vi "MakeArray.vi"(6 "Hviletid(s)":dbl, 9 "Amplitude(kPA)":dbl, 10 "Frekvens(kHz)":dbl, 11 "Temperatur(Celsius)":dbl) -> (3 "Array":dbl[](array[numeric]))   [LabVIEW 2015]
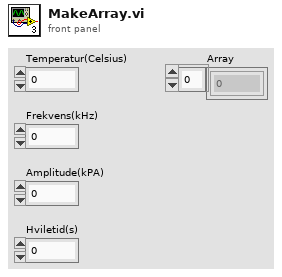
[diagram p1: front panel]
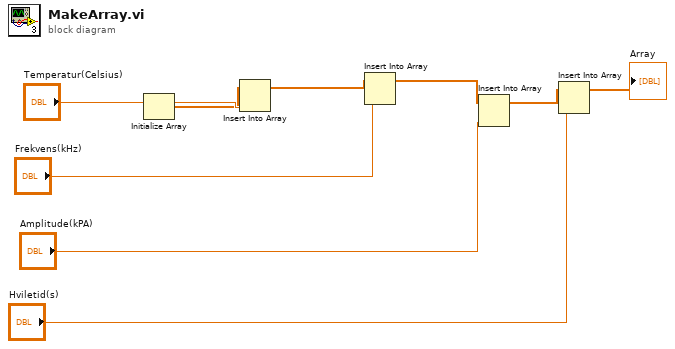
[diagram p0: block diagram]
diagram:
  n1 = Initialize Array("Temperatur(Celsius)") -> (w1:dbl[])  [unwired: 1 in]
  n2 = Insert Into Array(array=w1, new element="Temperatur(Celsius)") -> (w6:dbl[])  [unwired: 1 in]
  n3 = Insert Into Array(array=w6, new element="Frekvens(kHz)") -> (w7:dbl[])  [unwired: 1 in]
  n4 = Insert Into Array(array=w7, new element="Amplitude(kPA)") -> (w8:dbl[])  [unwired: 1 in]
  n5 = Insert Into Array(array=w8, new element="Hviletid(s)") -> (→"Array":dbl[])  [unwired: 1 in]
